vi "Get LabVIEW Files.vi"(8 "Error In":errorcluster, 11 "Revert Config":T1={"Revert Paths"={"Archive Path"=path "D:/workspace/revert/todo/todo.zip", "Unzip Directory"=path "D:/workspace/revert/unzip", "Backsave Directory"=path "D:/workspace/revert/backsave", "Output Archive"=path "D:/workspace/revert/backsave", "Backsave Common Directory"=path "D:/workspace/revert/backsave"}, "LabVIEW Files"={"Projects"=[], "Libraries"=[], "Classes"=[], "XControls"=[], "VIs and Controls"=[], "Non LV Files"=[]}, "LabVIEW Version"=enum."8.0"}) -> (0 "Error Out":errorcluster, 3 "Revert Config":T1={"Revert Paths"={"Archive Path"=path "D:/workspace/revert/todo/todo.zip", "Unzip Directory"=path "D:/workspace/revert/unzip", "Backsave Directory"=path "D:/workspace/revert/backsave", "Output Archive"=path "D:/workspace/revert/backsave", "Backsave Common Directory"=path "D:/workspace/revert/backsave"}, "LabVIEW Files"={"Projects"=[], "Libraries"=[], "Classes"=[], "XControls"=[], "VIs and Controls"=[], "Non LV Files"=[]}, "LabVIEW Version"=enum."8.0"})   [LabVIEW 2013, in "LVH-Revert.lvlib"]
uses:
  <vilib>/LabVIEW Hacker/Revert/LVH-Revert.lvlib
  <vilib>/LabVIEW Hacker/Revert/Type Defs/Revert Config.ctl
  <vilib>/LabVIEW Hacker/Revert/Type Defs/Paths.ctl
  <vilib>/LabVIEW Hacker/Revert/Type Defs/LabVIEW Files.ctl
  <vilib>/LabVIEW Hacker/LVH-Toolbox/Common/Private/Type Defs/LabVIEW Version.ctl
  <vilib>/LabVIEW Hacker/LVH-Toolbox/Common/LVH-Common.lvlib
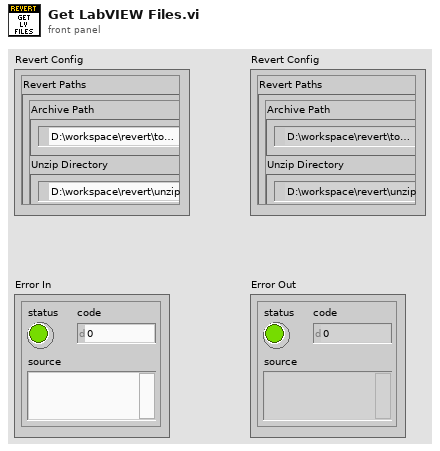
[diagram p1: front panel]
types:
  T1 = typedef "LVH-Revert.lvlib/Revert Config.ctl" = cluster{"Revert Paths":T2, "LabVIEW Files":T3, "LabVIEW Version":T4}
  T2 = typedef "LVH-Revert.lvlib/Paths.ctl" = cluster{"Archive Path":path, "Unzip Directory":path, "Backsave Directory":path, "Output Archive":path, "Backsave Common Directory":path}
  T3 = typedef "LVH-Revert.lvlib/LabVIEW Files.ctl" = cluster{"Projects":path[], "Libraries":path[], "Classes":path[], "XControls":path[], "VIs and Controls":path[], "Non LV Files":path[]}
  T4 = typedef "LVH-Toolbox.lvlib/LVH-Common.lvlib/LabVIEW Version.ctl" = enum16{"8.0", "8.2", "8.6", "9.0", "10.0", "11.0", "12.0", "13.0"}
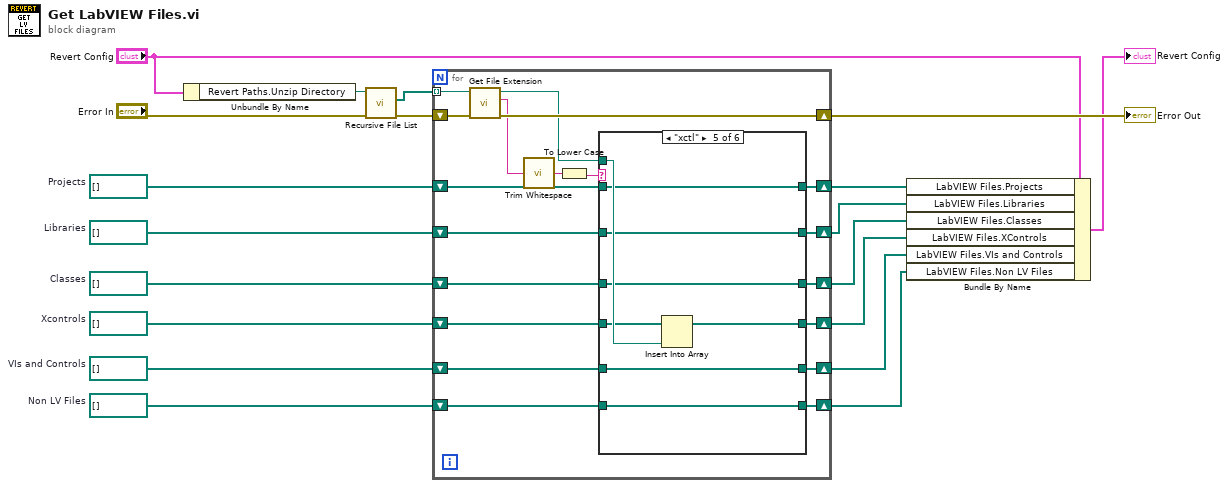
[diagram p0: block diagram]
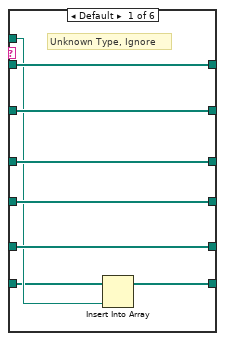
[diagram p2: hidden frame]
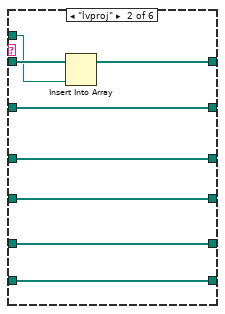
[diagram p3: hidden frame]
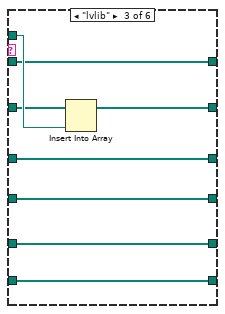
[diagram p4: hidden frame]
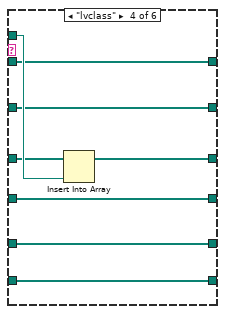
[diagram p5: hidden frame]
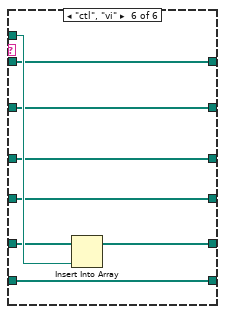
[diagram p6: hidden frame]
diagram:
  w2 = path[] []  # Non LV Files
  w16 = path[] []  # VIs and Controls
  w15 = path[] []  # Xcontrols
  w17 = path[] []  # Classes
  w18 = path[] []  # Libraries
  w19 = path[] []  # Projects
  n1 = Unbundle By Name("Revert Config") -> ("Revert Paths.Unzip Directory"=w8:path)
  n2 = call <vilib>:"Recursive File List.vi"("error in (no error)"="Error In", "Folder Path"=w8) -> ("error out"=w6:errorcluster, "All Files in Dir"=w5:path[])  [unwired: 5 in, 3 out]
  n3 = for {
    shift-right: [w37] -> w9
    shift-left: w6 -> [w38]
    shift-right: [w36] -> w14
    shift-left: w19 -> [w35]
    shift-right: [w34] -> w13
    shift-left: w18 -> [w33]
    shift-right: [w32] -> w12
    shift-left: w17 -> [w31]
    shift-right: [w30] -> w11
    shift-left: w15 -> [w29]
    shift-right: [w28] -> w10
    shift-left: w16 -> [w27]
    tunnel: w5 -> [w22] mode=indexing
    shift-right: [w20] -> w1
    shift-left: w2 -> [w21]
    n4 = call <vilib>:"Get File Extension.vi"("Error In"=w38, "File Path Control"=w22) -> ("Error Out"=w37:errorcluster, "Extension"=w24:string, "Duplicate Path"=w26:path)  [unwired: 7 in]
    n5 = call <vilib>:"Trim Whitespace.vi"("string"=w24) -> ("trimmed string"=w25:string)  [unwired: 1 in]
    n6 = To Lower Case(string=w25) -> (all lower case string=w23:string)
    n7 = case shown="\"xctl\"" w23 {
      tunnel: [w46 w52 w56 w67 w76 w85] -> w36
      tunnel: w35 -> [w46 w54 w56 w67 w76 w85]
      tunnel: [w45 w51 w57 w66 w75 w84] -> w34
      tunnel: w33 -> [w45 w51 w58 w66 w75 w84]
      tunnel: [w44 w50 w61 w64 w74 w83] -> w32
      tunnel: w31 -> [w44 w50 w61 w65 w74 w83]
      tunnel: [w43 w49 w60 w69 w72 w80] -> w30
      tunnel: w29 -> [w43 w49 w60 w69 w73 w80]
      tunnel: [w42 w48 w59 w68 w77 w81] -> w28
      tunnel: w27 -> [w42 w48 w59 w68 w77 w82]
      tunnel: w26 -> [w41 w53 w62 w70 w78 w86]
      tunnel: w21 -> [w39 w47 w55 w63 w71 w79]
      tunnel: [w40 w47 w55 w63 w71 w79] -> w20
      frame Default {
        # "Unknown Type, Ignore"
        n8 = Insert Into Array(array=w39, new element=w41) -> (w40:path[])  [unwired: 1 in]
      }
      frame "lvproj" {
        n9 = Insert Into Array(array=w54, new element=w53) -> (w52:path[])  [unwired: 1 in]
      }
      frame "lvlib" {
        n10 = Insert Into Array(array=w58, new element=w62) -> (w57:path[])  [unwired: 1 in]
      }
      frame "lvclass" {
        n11 = Insert Into Array(array=w65, new element=w70) -> (w64:path[])  [unwired: 1 in]
      }
      frame "xctl" {
        n12 = Insert Into Array(array=w73, new element=w78) -> (w72:path[])  [unwired: 1 in]
      }
      frame "ctl", "vi" {
        n13 = Insert Into Array(array=w82, new element=w86) -> (w81:path[])  [unwired: 1 in]
      }
    }
  }
  "Error Out" <- w9
  n14 = Bundle By Name(cluster="Revert Config", "LabVIEW Files.Projects"=w14, "LabVIEW Files.Libraries"=w13, "LabVIEW Files.Classes"=w12, "LabVIEW Files.XControls"=w11, "LabVIEW Files.VIs and Controls"=w10, "LabVIEW Files.Non LV Files"=w1) -> (→"Revert Config":T1)
